vi "Test Get Cell (String).vi"(11 "Test Case In":refnum<class "Test Open Xml.lvclass">) -> (0 "error out":errorcluster, 3 "Test Case Out":refnum<class "Test Open Xml.lvclass">)   [LabVIEW 2021, in "Test Open Xml.lvclass"]
uses:
  Test Open Xml.lvclass
  C:/Program Files/National Instruments/LabVIEW 2025/vi.lib/Astemes/LUnit/Test Case.lvclass
  <vilib>/Astemes/LUnit/Test Case.lvclass/Test Case.ctl
  e7d09ce7-04db-40ce-9c4e-a78b31ec9fe8.vi
  <vilib>/Astemes/LUnit/Core/LUnit Test Case/Private/Append Pass Result.vi
  <vilib>/Astemes/LUnit/Core/LUnit Test Case/Private/Append Fail Result.vi
  e7d09ce7-04db-40ce-9c4e-a78b31ec9fe8.vi/9c5d11cd-9439-4240-a1ee-d9baace9c924.vi
  <vilib>/Astemes/LUnit/Core/LUnit Test Case/Private/Run In UI.vi
  <vilib>/Utility/error.llb/Clear Errors.vi
  Source/Open Xml.lvlib
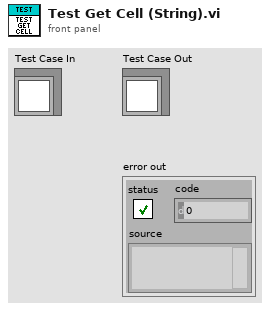
[diagram p1: front panel]
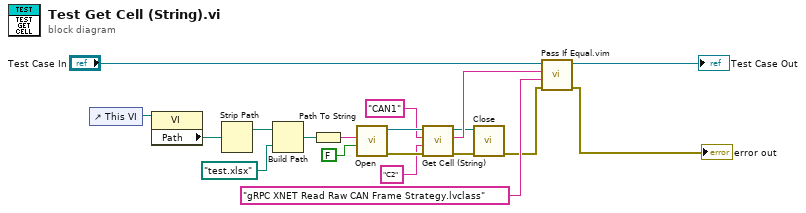
[diagram p0: block diagram]
diagram:
  n1 = control-ref of="This VI"() -> (w16:refnum<vi>)
  n2 = property class="VI"(reference=w16) -> ("Path"=w15:path)  [unwired: 1 in, 2 out]
  n3 = Strip Path(path=w15) -> (stripped path=w14:path)  [unwired: 1 out]
  n4 = Build Path(base path=w14, name or relative path=path "test.xlsx") -> (appended path=w12:path)
  n5 = Path To String(path=w12) -> (string=w11:string)
  n6 = call "Open.vi"("isEditable"=FALSE, "Path"=w11) -> ("error out"=w8:errorcluster, "SpreadsheetDocument"=w9:refnum<k24>)  [unwired: 8 in]
  n7 = call "Get Cell (String).vi"("error in"=w8, "Cell Address"="C2", "Sheet Name"="CAN1", "SpreadsheetDocument"=w9) -> ("error out"=w3:errorcluster, "Value String"=w5:string, "SpreadsheetDocument out"=w1:refnum<k24>)  [unwired: 5 in]
  n8 = call "Close.vi"("error in"=w3, "SpreadsheetDocument"=w1) -> ("error out"=w2:errorcluster)  [unwired: 9 in]
  n9 = call "Pass If Equal.vim"("error in (no error)"=w2, "Actual"="gRPC XNET Read Raw CAN Frame Strategy.lvclass", "Expected"=w5, "LUnit Test Case In"="Test Case In") -> ("error out"=→"error out":errorcluster, "LUnit Test Case Out"=→"Test Case Out":refnum<class "Test Open Xml.lvclass">)  [unwired: 6 in]
